vi "Get Velocity.vi"(8 "error in (no error)":errorcluster, 11 "DC Motor Controller Sim in":refnum<class "DC Motor Controller Simulator.lvclass">) -> (0 "error out":errorcluster, 2 "CCW Velocity (rad/s)":dbl, 3 "DC Motor Controller Sim out":refnum<class "DC Motor Controller Simulator.lvclass">)   [LabVIEW 2019, in "DC Motor Controller Simulator.lvclass"]
doc: "Queries the counterclockwise velocity from the motor encoder."
uses:
  DC Motor Controller Simulator.lvclass
  <vilib>/robotics/Simulator/Robot Factory/Motor/ODESimulator_Motor.lvclass
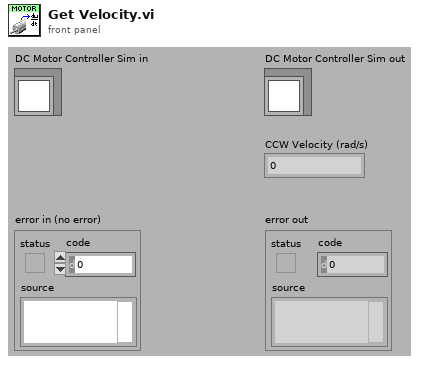
[diagram p1: front panel]
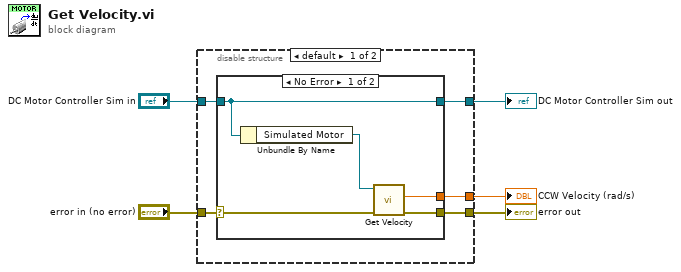
[diagram p0: block diagram]
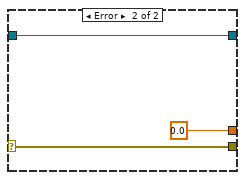
[diagram p2: hidden frame]
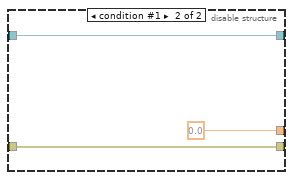
[diagram p3: hidden frame]
diagram:
  n1 = disable-structure shown="default" {
    disable-tunnel: "error in (no error)" -> [w10 w20]
    disable-tunnel: "DC Motor Controller Sim in" -> [w9 w21]
    disable-tunnel: [w8 w21] -> w2
    disable-tunnel: [w7 w20] -> w1
    disable-tunnel: [w6 0.0] -> w3
    frame condition #0 (active) {
      n2 = case shown="No Error" w10 {
        selector: w10 -> [w13 w17]
        tunnel: w9 -> [w15 w18]
        tunnel: [w15 w18] -> w8
        tunnel: [w12 w17] -> w7
        tunnel: [w11 0.0] -> w6
        frame No Error {
          n3 = Unbundle By Name(w15) -> ("Simulated Motor"=w14:refnum<class "ODESimulator_Motor.lvclass">)
          n4 = call-dynamic "Get Velocity.vi"("error in (no error)"=w13, "Motor in"=w14) -> ("error out"=w12:errorcluster, "CCW Velocity (rad/s)"=w11:dbl)  [unwired: 7 in, 1 out]
        }
        frame Error {
        }
      }
    }
    frame condition #1 {
    }
  }
  "error out" <- w1
  "DC Motor Controller Sim out" <- w2
  "CCW Velocity (rad/s)" <- w3
